vi "NISE.Open Physical Channel Command.vi"(0 "SLSC Interface in":refnum<class "SLSC Interface.lvclass">, 5 "physical channel":refnum<k21>="$DefaultPhysChans", 7 "command in":refnum<k21>, 11 "error in (no error)":errorcluster) -> (4 "SLSC Interface out":refnum<class "SLSC Interface.lvclass">, 8 "command out":refnum<k21>, 15 "error out":errorcluster)   [LabVIEW 2016, in "SLSC Interface.lvclass"]
uses:
  SLSC Interface.lvclass
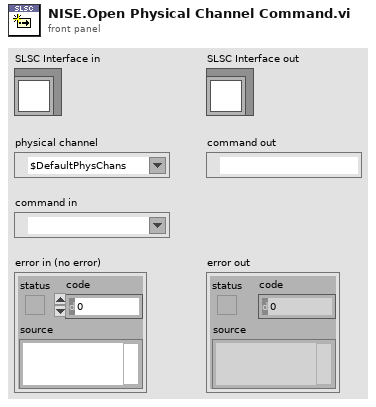
[diagram p1: front panel]
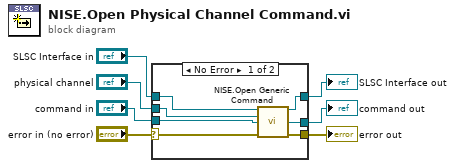
[diagram p0: block diagram]
diagram:
  n1 = case shown="No Error" "error in (no error)" {
    selector: "error in (no error)" -> [w12 w16]
    tunnel: [w11 w16] -> w6
    tunnel: [w13 w15] -> w4
    tunnel: "SLSC Interface in" -> [w14 w15]
    tunnel: "physical channel" -> [w10 _]
    tunnel: [w9 _] -> w2
    tunnel: "command in" -> [w8 _]
    frame No Error {
      n2 = call "NISE.Open Generic Command.vi"("SLSC Interface in"=w14, "resource"=w10, "command in"=w8, "error in (no error)"=w12) -> ("SLSC Interface out"=w13:refnum<class "SLSC Interface.lvclass">, "command out"=w9:refnum<k21>, "error out"=w11:errorcluster)  [unwired: 9 in]
    }
    frame Error {
    }
  }
  "error out" <- w6
  "SLSC Interface out" <- w4
  "command out" <- w2
